vi "Vision 표지판 인식.vi"() -> ()   [LabVIEW 2016]
uses:
  <vilib>/vision/Classification.llb/IMAQ Classifier Nearest Neighbor options.ctl
  <vilib>/vision/NI_Vision_Development_Module.lvlib
  <vilib>/ptbypt/NI_PtbyPt.lvlib
panel:
  out "횡단보도 거리":dbl[](array[numeric])
  in  "탭 컨트롤 3":enum32{"유턴", "동적", "정적"}(tab)
  out "유턴":T1(plugin-control)
  out "동적":T1(plugin-control)
  out "정적":T1(plugin-control)
  in  "탭 컨트롤 2":enum32{"유턴", "동적", "정적"}(tab)
  in  "File Path":path=path "C:/Users/SeongHyeon/Desktop/전체프로그램/Sub Vi/Sensor/Vision Reference/유턴.clf"
  in  "File Path 2":path=path "C:/Users/SeongHyeon/Desktop/전체프로그램/Sub Vi/Sensor/Vision Reference/동적.clf"
  in  "File Path 3":path=path "C:/Users/SeongHyeon/Desktop/전체프로그램/Sub Vi/Sensor/Vision Reference/정적.clf"
  in  "탭 컨트롤":enum32{"유턴", "동적", "정적"}(tab)
  in  "Paramaters":T3={"Preprocessing Options"={"Method"=-1, "Looking for"=1, "Threshold Range"={"Lower value"=0.0, "Upper value"=31.0}, "Threshold Limits"={"Lower value"=0.0, "Upper value"=0.0}, "Reject Border"=FALSE, "# of Erosions"=0, "Kernel Size"={"Lower value"=0, "Upper value"=0}, "Deviation Factor"=0.0}, "Nearest Neighbor Options"={"Method"=0, "Metric"=0, "k"=0}, "Particle Options"={"Scale Dependant"=FALSE, "Scale Factor"=0.0, "Symmetry Dependant"=FALSE, "Symmetry Factor"=0.0}} {"Preprocessing Options"."Deviation Factor" min=0.0; "Preprocessing Options"."Threshold Limits"."Upper value" format="%.2f"; "Preprocessing Options"."Threshold Limits"."Lower value" format="%.2f"; "Preprocessing Options"."Threshold Range"."Upper value" format="%.2f"; "Preprocessing Options"."Threshold Range"."Lower value" format="%.2f"; "Preprocessing Options"."# of Erosions" min=0; "Preprocessing Options"."Method" items=["Manual Threshold"=-1, "-"=-2, "Auto Threshold: Clustering"=0, "Auto Threshold: Entropy"=1, "Auto Threshold: Metric"=2, "Auto Threshold: Moments"=3, "Auto Threshold: Inter-class Variance"=4, "--"=-3, "Local Threshold: Niblack"=5, "Local Threshold: BG Correction"=6]; "Preprocessing Options"."Looking for" items=["Bright Objects", "Dark Objects"]; "Nearest Neighbor Options"."Method" items=["Nearest Neighbor", "K Nearest Neighbor", "Minimum Mean Distance"]; "Nearest Neighbor Options"."Metric" items=["Maximum", "Sum", "Euclidean"]; "Nearest Neighbor Options"."k" min=3}
  in  "Paramaters 2":T3={"Preprocessing Options"={"Method"=-1, "Looking for"=0, "Threshold Range"={"Lower value"=0.0, "Upper value"=45.0}, "Threshold Limits"={"Lower value"=0.0, "Upper value"=0.0}, "Reject Border"=FALSE, "# of Erosions"=0, "Kernel Size"={"Lower value"=0, "Upper value"=0}, "Deviation Factor"=0.0}, "Nearest Neighbor Options"={"Method"=0, "Metric"=0, "k"=0}, "Particle Options"={"Scale Dependant"=FALSE, "Scale Factor"=0.0, "Symmetry Dependant"=FALSE, "Symmetry Factor"=0.0}} {"Preprocessing Options"."Deviation Factor" min=0.0; "Preprocessing Options"."Threshold Limits"."Upper value" format="%.2f"; "Preprocessing Options"."Threshold Limits"."Lower value" format="%.2f"; "Preprocessing Options"."Threshold Range"."Upper value" format="%.2f"; "Preprocessing Options"."Threshold Range"."Lower value" format="%.2f"; "Preprocessing Options"."# of Erosions" min=0; "Preprocessing Options"."Method" items=["Manual Threshold"=-1, "-"=-2, "Auto Threshold: Clustering"=0, "Auto Threshold: Entropy"=1, "Auto Threshold: Metric"=2, "Auto Threshold: Moments"=3, "Auto Threshold: Inter-class Variance"=4, "--"=-3, "Local Threshold: Niblack"=5, "Local Threshold: BG Correction"=6]; "Preprocessing Options"."Looking for" items=["Bright Objects", "Dark Objects"]; "Nearest Neighbor Options"."Method" items=["Nearest Neighbor", "K Nearest Neighbor", "Minimum Mean Distance"]; "Nearest Neighbor Options"."Metric" items=["Maximum", "Sum", "Euclidean"]; "Nearest Neighbor Options"."k" min=3}
  in  "Paramaters 3":T3={"Preprocessing Options"={"Method"=-1, "Looking for"=0, "Threshold Range"={"Lower value"=0.0, "Upper value"=45.0}, "Threshold Limits"={"Lower value"=0.0, "Upper value"=0.0}, "Reject Border"=FALSE, "# of Erosions"=0, "Kernel Size"={"Lower value"=0, "Upper value"=0}, "Deviation Factor"=0.0}, "Nearest Neighbor Options"={"Method"=0, "Metric"=0, "k"=0}, "Particle Options"={"Scale Dependant"=FALSE, "Scale Factor"=0.0, "Symmetry Dependant"=FALSE, "Symmetry Factor"=0.0}} {"Preprocessing Options"."Deviation Factor" min=0.0; "Preprocessing Options"."Threshold Limits"."Upper value" format="%.2f"; "Preprocessing Options"."Threshold Limits"."Lower value" format="%.2f"; "Preprocessing Options"."Threshold Range"."Upper value" format="%.2f"; "Preprocessing Options"."Threshold Range"."Lower value" format="%.2f"; "Preprocessing Options"."# of Erosions" min=0; "Preprocessing Options"."Method" items=["Manual Threshold"=-1, "-"=-2, "Auto Threshold: Clustering"=0, "Auto Threshold: Entropy"=1, "Auto Threshold: Metric"=2, "Auto Threshold: Moments"=3, "Auto Threshold: Inter-class Variance"=4, "--"=-3, "Local Threshold: Niblack"=5, "Local Threshold: BG Correction"=6]; "Preprocessing Options"."Looking for" items=["Bright Objects", "Dark Objects"]; "Nearest Neighbor Options"."Method" items=["Nearest Neighbor", "K Nearest Neighbor", "Minimum Mean Distance"]; "Nearest Neighbor Options"."Metric" items=["Maximum", "Sum", "Euclidean"]; "Nearest Neighbor Options"."k" min=3}
  out "정적이냐":bool
  out "동적이냐":bool
  in  "ID":enum32{"External", "Internal"}(ring)
  in  "Type":u32(ring)=3 items=["No Selection", "Point", "Line", "Rectangle", "Oval", "Polygon", "Free", "Annulus", "Unused2", "Unused3", "Broken Line", "Free Hand Line", "Rotated Rectangle"]
  out "유턴이냐":bool
  in  "Stop (F)":bool
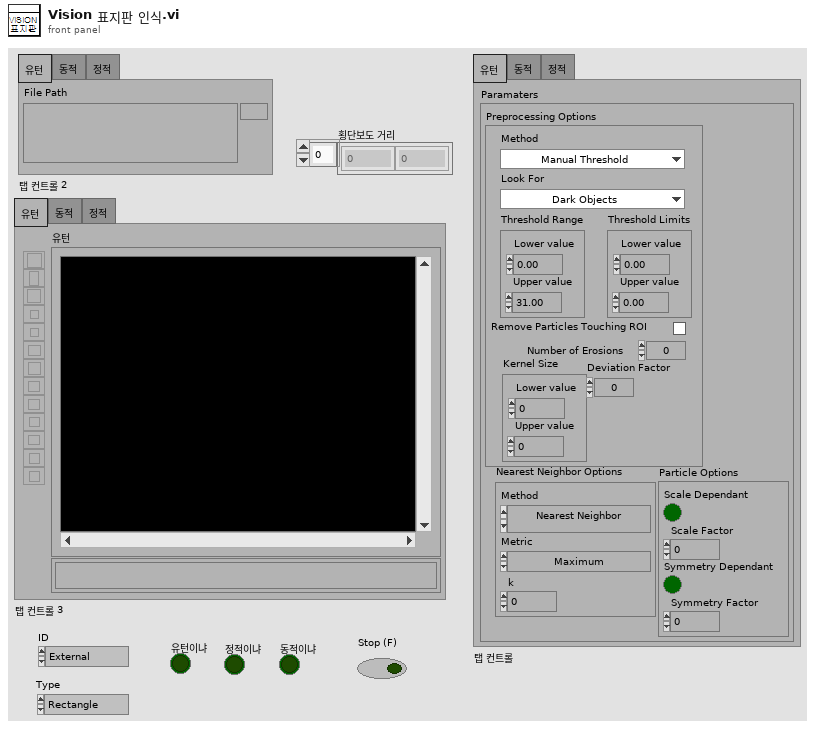
[diagram p1: front panel]
types:
  T1 = typedef "IMAQ Image.ctl" = refnum<image>
  T2 = typedef "IMAQ Classifier Nearest Neighbor options.ctl" = cluster{"Method":i32, "Metric":i32, "k":i32}
  T3 = cluster{"Preprocessing Options":cluster{"Method":i32, "Looking for":i32, "Threshold Range":cluster{"Lower value":sgl, "Upper value":sgl}, "Threshold Limits":cluster{"Lower value":sgl, "Upper value":sgl}, "Reject Border":bool, "# of Erosions":i32, "Kernel Size":cluster{"Lower value":i32, "Upper value":i32}, "Deviation Factor":dbl}, "Nearest Neighbor Options":T2, "Particle Options":cluster{"Scale Dependant":bool, "Scale Factor":sgl, "Symmetry Dependant":bool, "Symmetry Factor":sgl}}
  T4 = typedef "Image Type" = u32
  T5 = cluster{"Global Rectangle":cluster{"x1Left":i32, "y1Top":i32, "x2Right":i32, "y2Bottom":i32}, "Centroid":cluster{"x":sgl, "y":sgl}, "Object Size":u32, "Score":dbl}[]
  T6 = cluster{"Position":cluster{"x":sgl, "y":sgl}, "Angle":sgl, "Scale":sgl, "Score":sgl, "Bounding Box":cluster{"x":sgl, "y":sgl}[]}[]
  T7 = cluster{"Position":cluster{"x":sgl, "y":sgl}, "Angle":sgl, "Scale":sgl, "Score":sgl, "Bounding Box":cluster{"x":sgl, "y":sgl}[]}
  T8 = cluster{"Global Rectangle":cluster{"x1Left":i32, "y1Top":i32, "x2Right":i32, "y2Bottom":i32}, "Centroid":cluster{"x":sgl, "y":sgl}, "Object Size":u32, "Score":dbl}
  T9 = cluster{"x1Left":i32, "y1Top":i32, "x2Right":i32, "y2Bottom":i32}
  T10 = cluster{"ID":enum32{"External", "Internal"}, "Type":u32, "Global Rectangle":i32[]}
  T11 = cluster{"ID":enum32{"External", "Internal"}, "Type":u32, "Global Rectangle":i32[]}[]
  T12 = cluster{"Global Rectangle":i32[], cluster{"ID":enum32{"External", "Internal"}, "Type":u32, "Global Rectangle":i32[]}[]}
  T13 = typedef "IMAQ Classifier Session.ctl" = refnum<k1>
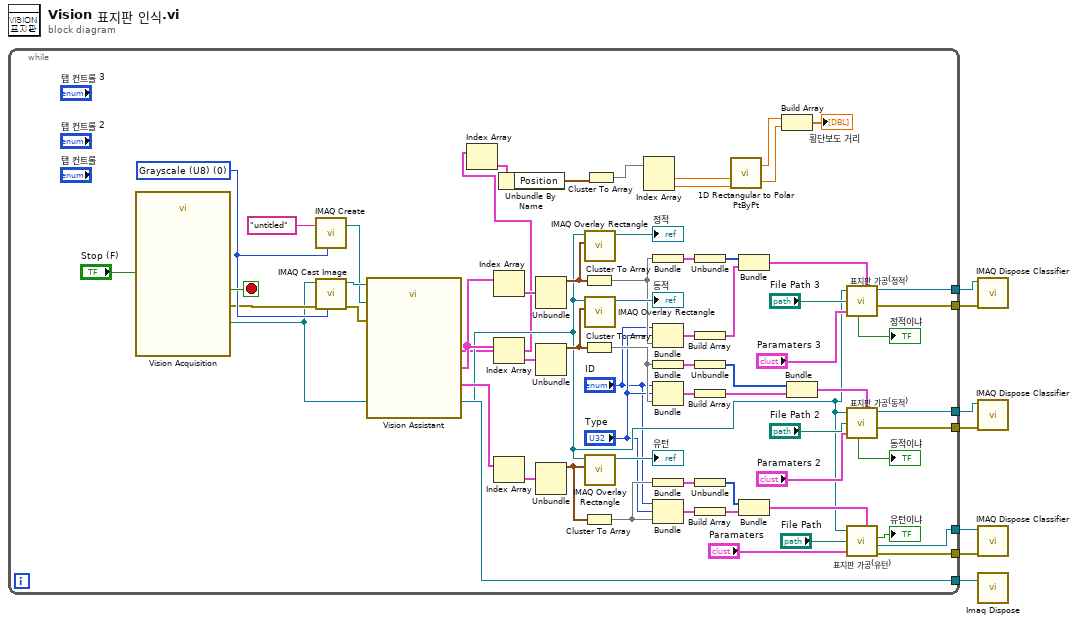
[diagram p0: block diagram]
diagram:
  n1 = while {
    tunnel: [w58] -> w7
    tunnel: [w50] -> w6
    tunnel: [w37] -> w5
    tunnel: [w36] -> w4
    tunnel: [w35] -> w3
    tunnel: [w23] -> w2
    tunnel: [w22] -> w1
    stop <- w71 stop-if-true
    w69 = T4 0 items=["Grayscale (U8)", "Grayscale (I16)", "Grayscale (SGL)", "Complex (CSG)", "RGB (U32)", "HSL (U32)", "RGB (U64)", "Grayscale (U16)"] ("Image Type")
    n2 = call "Vision Acquisition"("Stop (F)"="Stop (F)") -> ("Image Out"=w19:T1, "Stopped"=w71:bool, "error out"=w65:errorcluster)  [unwired: 24 in]
    n3 = call "IMAQ Create"("Image Name"="untitled", "Image Type"=w69) -> ("New Image"=w55:T1)  [unwired: 3 in, 1 out]
    n4 = call "IMAQ Cast Image"("Image Type"=w69, "error in (no error)"=w65, "Image Src"=w19) -> ("error out"=w66:errorcluster, "Image Dst Out"=w56:T1)  [unwired: 7 in]
    n5 = call "Vision Assistant"("Image In"=w56, "Image Dst"=w55, "error in"=w66) -> ("Image Out"=w58:T1, "Shape Report (calibrated) (Shape Matching 1)"=w68:T5, "Shape Report (Shape Matching 2)"=w24:T5, "Calibrated Matches (Pattern Matching 1)"=w8:T6)  [unwired: 20 in, 1 out]
    n6 = Index Array(array=w8) -> (element=w16:T7)  [unwired: 1 in]
    n7 = Index Array(array=w24) -> (element=w32:T8)  [unwired: 1 in]
    n8 = Index Array(array=w24) -> (element=w49:T8)  [unwired: 1 in]
    n9 = Index Array(array=w68) -> (element=w67:T8)  [unwired: 1 in]
    n10 = Unbundle By Name(w16) -> ("Position"=w15:cluster{"x":sgl, "y":sgl})
    n11 = Unbundle(w32) -> ("Global Rectangle"=w25:T9)  [unwired: 3 out]
    n12 = Unbundle(w49) -> ("Global Rectangle"=w42:T9)  [unwired: 3 out]
    n13 = Unbundle(w67) -> ("Global Rectangle"=w57:T9)  [unwired: 3 out]
    n14 = Cluster To Array(cluster=w25) -> (array=w31:i32[])
    n15 = Cluster To Array(cluster=w42) -> (array=w48:i32[])
    n16 = Cluster To Array(cluster=w57) -> (array=w64:i32[])
    n17 = call "IMAQ Overlay Rectangle"("Rectangle"=w25, "Image"=w19) -> ("Image Out"=→"정적":T1)  [unwired: 8 in, 1 out]
    n18 = call "IMAQ Overlay Rectangle"("Rectangle"=w42, "Image"=w19) -> ("Image Out"=→"동적":T1)  [unwired: 8 in, 1 out]
    n19 = call "IMAQ Overlay Rectangle"("Rectangle"=w57, "Image"=w19) -> ("Image Out"=→"유턴":T1)  [unwired: 8 in, 1 out]
    n20 = Cluster To Array(cluster=w15) -> (array=w14:sgl[])
    n21 = Index Array(array=w14) -> (element #1=w13:sgl, element #2=w12:sgl)  [unwired: 2 in]
    n22 = Bundle("Global Rectangle"=w31) -> (w30:cluster{"Global Rectangle":i32[]})  [unwired: 1 in]
    n23 = Bundle("ID"="ID", "Type"="Type", "Global Rectangle"=w31) -> (w28:T10)  [unwired: 1 in]
    n24 = Bundle("Global Rectangle"=w48) -> (w47:cluster{"Global Rectangle":i32[]})  [unwired: 1 in]
    n25 = Bundle("ID"="ID", "Type"="Type", "Global Rectangle"=w48) -> (w45:T10)  [unwired: 1 in]
    n26 = Bundle("Global Rectangle"=w64) -> (w63:cluster{"Global Rectangle":i32[]})  [unwired: 1 in]
    n27 = Bundle("ID"="ID", "Type"="Type", "Global Rectangle"=w64) -> (w61:T10)  [unwired: 1 in]
    n28 = Unbundle(w30) -> ("Global Rectangle"=w29:i32[])
    n29 = Build Array(w28) -> (w27:T11)
    n30 = Unbundle(w47) -> ("Global Rectangle"=w46:i32[])
    n31 = Build Array(w45) -> (w44:T11)
    n32 = Unbundle(w63) -> ("Global Rectangle"=w62:i32[])
    n33 = Build Array(w61) -> (w60:T11)
    n34 = call <vilib>:"1D Rectangular to Polar PtByPt.vi"("y"=w12, "x"=w13) -> ("phase"=w10:dbl, "magnitude"=w11:dbl)
    n35 = Bundle("Global Rectangle"=w29, w27) -> (w20:T12)  [unwired: 1 in]
    n36 = Bundle("Global Rectangle"=w62, w60) -> (w52:T12)  [unwired: 1 in]
    n37 = Build Array(w11, w10) -> (→"횡단보도 거리":dbl[])
    n38 = Bundle("Global Rectangle"=w46, w44) -> (w39:T12)  [unwired: 1 in]
    n39 = call "표지판 가공(정적).vi"("Image 2"=w19, "File Path"="File Path 3", "Paramaters"="Paramaters 3", "ROI Descriptor (Particle Classification 1)"=w20) -> ("주차냐"=→"정적이냐":bool, "Classifier Session (dup)"=w23:T13, "error out"=w22:errorcluster)  [unwired: 3 in, 1 out]
    n40 = call "표지판 가공(동적).vi"("Image 2"=w19, "File Path"="File Path 2", "Paramaters"="Paramaters 2", "ROI Descriptor (Particle Classification 1)"=w39) -> ("주차냐"=→"동적이냐":bool, "Classifier Session (dup)"=w37:T13, "error out"=w35:errorcluster)  [unwired: 3 in, 1 out]
    n41 = call "표지판 가공(유턴).vi"("Image 2"=w19, "File Path"="File Path", "Paramaters"="Paramaters", "ROI Descriptor (Particle Classification 1)"=w52) -> ("주차냐"=→"유턴이냐":bool, "Classifier Session (dup)"=w50:T13, "error out"=w36:errorcluster)  [unwired: 3 in, 1 out]
  }
  n42 = call "IMAQ Dispose Classifier"("error in (no error)"=w1, "Classifier Session"=w2) -> ()  [unwired: 9 in, 1 out]
  n43 = call "IMAQ Dispose Classifier"("error in (no error)"=w3, "Classifier Session"=w5) -> ()  [unwired: 9 in, 1 out]
  n44 = call "IMAQ Dispose Classifier"("error in (no error)"=w4, "Classifier Session"=w6) -> ()  [unwired: 9 in, 1 out]
  n45 = call "Imaq Dispose"("Image"=w7) -> ()  [unwired: 5 in, 1 out]
